vi "time.vi"(1 "# seconds":dbl, 2 "digit precision (6)":i16) -> (8 "Reduced Time":string)   [LabVIEW 2017]
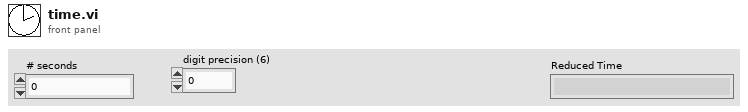
[diagram p1: front panel]
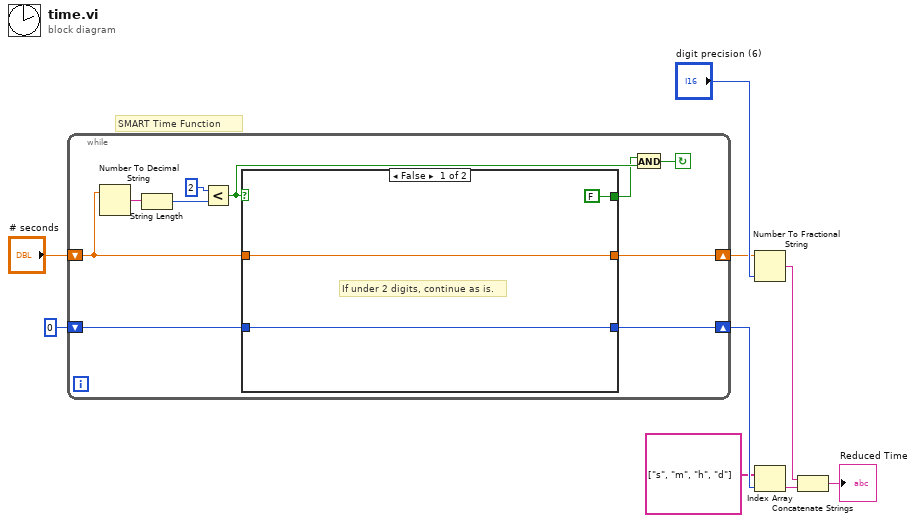
[diagram p0: block diagram]
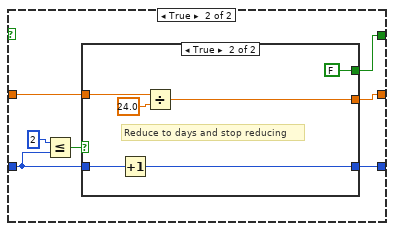
[diagram p2: hidden frame]
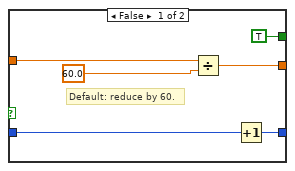
[diagram p3: hidden frame]
diagram:
  # "SMART Time Function"
  n1 = while {
    shift-right: [w15] -> w3
    shift-left: "# seconds" -> [w16]
    shift-right: [w10] -> w5
    shift-left: 0 -> [w11]
    stop <- w14 continue-if-true
    n2 = Number To Decimal String(number=w16) -> (decimal integer string=w19:string)  [unwired: 1 in]
    n3 = String Length(string=w19) -> (length=w18:i32)
    n4 = Less?(x=2, y=w18) -> (x < y?=w13:bool)
    n5 = case shown="False" w13 {
      tunnel: w16 -> [w22 w27]
      tunnel: [w22 w26] -> w15
      tunnel: [FALSE w25] -> w12
      tunnel: w11 -> [w20 w24]
      tunnel: [w20 w23] -> w10
      frame False {
        # "If under 2 digits, continue as is."
      }
      frame True {
        n6 = Less Or Equal?(x=2, y=w24) -> (x <= y?=w29:bool)
        n7 = case shown="True" w29 {
          tunnel: w27 -> [w34 w40]
          tunnel: [w32 w39] -> w26
          tunnel: [TRUE FALSE] -> w25
          tunnel: w24 -> [w31 w37]
          tunnel: [w30 w36] -> w23
          frame False {
            # "Default: reduce by 60."
            n8 = Divide(x=w34, y=60.0) -> (x/y=w32:dbl)
            n9 = Increment(x=w31) -> (x+1=w30:i32)
          }
          frame True {
            # "Reduce to days and stop reducing"
            n10 = Increment(x=w37) -> (x+1=w36:i32)
            n11 = Divide(x=w40, y=24.0) -> (x/y=w39:dbl)
          }
        }
      }
    }
    n12 = And(x=w12, y=w13) -> (x .and. y?=w14:bool)
  }
  n13 = Number To Fractional String(number=w3, precision (6)="digit precision (6)") -> (F-format string=w7:string)  [unwired: 2 in]
  n14 = Index Array(array=string[] ["s", "m", "h", "d"], index=w5) -> (element=w6:string)
  n15 = Concatenate Strings(w7, w6) -> (→"Reduced Time":string)
